vi "MercuryIPSInit.vi"(1 "Inst bool":u64, 2 "Inst_param":T1) -> ()   [LabVIEW 2013]
uses:
  <instrlib>/Mercury iXX/Public/Controls/Comms Transport Layer.ctl
  <instrlib>/Mercury iXX/Public/Controls/Serial Settings.ctl
  <instrlib>/Mercury iXX/Public/Controls/ISOBus Address.ctl
  <instrlib>/Mercury iXX/Mercury iXX.lvlib
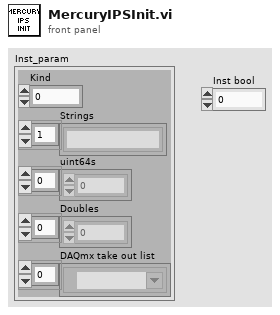
[diagram p1: front panel]
types:
  T1 = cluster{"Kind":u16, "Strings":string[], "uint64s":u64[], "Doubles":dbl[], "DAQmx take out list":refnum<k21>[]}
  T2 = typedef "Mercury iXX.lvlib/Comms Transport Layer.ctl" = enum16{"Ethernet TCP/IP", "USB", "ISOBus - RS-232", "GPIB"}
  T3 = typedef "Mercury iXX.lvlib/Serial Settings.ctl" = cluster{"Baud Rate":u32, "Parity":u16, "Data Bits":u16, "Stop Bits":u16, "Flow Control":u16}
  T4 = typedef "Mercury iXX.lvlib/ISOBus Address.ctl" = i32
  T5 = cluster{"VISA resource name":refnum<visa-resource-name>, "Comms Layer":T2, "IP Address":string, "Serial Configuration":T3, "ISOBUS address":T4}
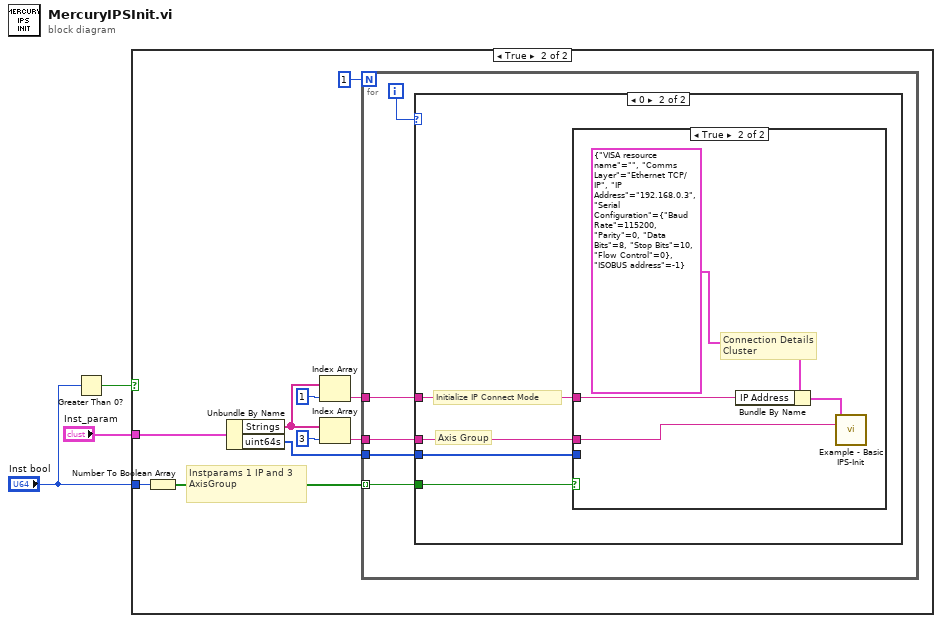
[diagram p0: block diagram]
diagram:
  n1 = Greater Than 0?(x="Inst bool") -> (x > 0?=w3:bool)
  n2 = case shown="True" w3 {
    tunnel: "Inst_param" -> [_ w13]
    tunnel: "Inst bool" -> [_ w11]
    frame False {
    }
    frame True {
      # "Instparams 1 IP and 3 AxisGroup"
      n3 = Number To Boolean Array(number=w11) -> (Boolean array=w10:bool[])
      n4 = Unbundle By Name(w13) -> ("Strings"=w5:string[], "uint64s"=w8:u64[])
      n5 = Index Array(array=w5, index=1) -> (element=w7:string)
      n6 = Index Array(array=w5, index=3) -> (element=w4:string)
      n7 = for {
        N: 1 -> [_]
        tunnel: w10 -> [w16] mode=indexing
        tunnel: w8 -> [w18]
        tunnel: w7 -> [w15]
        tunnel: w4 -> [w14]
        i -> [w17]
        n8 = case shown="0" w17 {
          tunnel: w18 -> [_ w21]
          tunnel: w16 -> [_ w22]
          tunnel: w15 -> [_ w20]
          tunnel: w14 -> [_ w19]
          frame 100, Default {
          }
          frame 0 {
            # "Axis Group"
            # "Initialize IP Connect Mode"
            n9 = case shown="True" w22 {
              tunnel: w21 -> [_ _]
              tunnel: w20 -> [_ w25]
              tunnel: w19 -> [_ w26]
              frame False {
              }
              frame True {
                # "Connection Details \nCluster"
                n10 = Bundle By Name(cluster=T5 {"VISA resource name"="", "Comms Layer"=enum."Ethernet TCP/IP", "IP Address"="192.168.0.3", "Serial Configuration"={"Baud Rate"=115200, "Parity"=0, "Data Bits"=8, "Stop Bits"=10, "Flow Control"=0}, "ISOBUS address"=-1} ("Connection Details"), "IP Address"=w25) -> (w23:T5)
                n11 = call <instrlib>:"Example - Basic IPS-Init.vi"("Connection Details"=w23, "Axis Group"=w26) -> ()  [unwired: 4 in, 10 out]
              }
            }
          }
        }
      }
    }
  }
